vi "Read.Lookup.vi"(8 "error in (no error)":errorcluster, 10 "Name":string, 11 "Data Access API in":refnum<class "Data Access Engine.lvclass">) -> (0 "error out":errorcluster, 1 "Found?":bool, 2 "Ref":refnum<data-value>, 3 "Data Access API out":refnum<class "Data Access Engine.lvclass">)   [LabVIEW 2015, in "Data Access Engine.lvlib" / "Data Access Engine.lvclass"]
uses:
  Data Access Engine.lvclass
  Data/Read/Read.lvclass
  Data Access Engine.lvclass/Data Access Engine.ctl
  Types/VS Channel Group Type.ctl
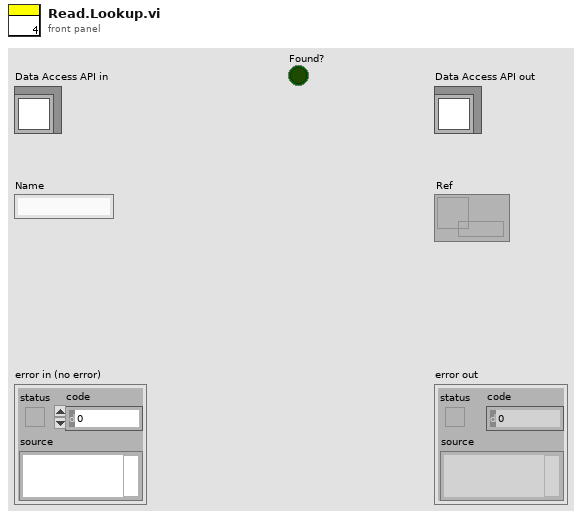
[diagram p1: front panel]
types:
  T1 = typedef "Data Access Engine.lvlib/Data Access Engine.lvclass/VS Channel Group Type.ctl" = enum16{"Output/Write", "Input/Read", "Input/ReadWrite"}
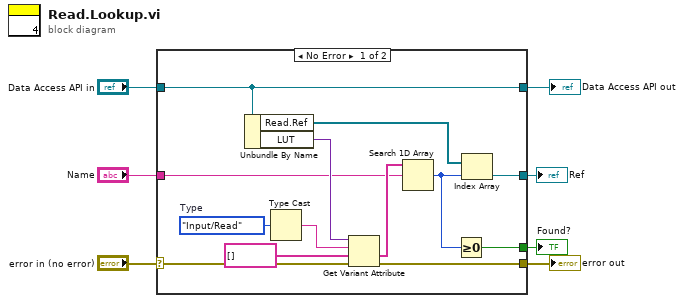
[diagram p0: block diagram]
diagram:
  n1 = case shown="No Error" "error in (no error)" {
    selector: "error in (no error)" -> [w16 w22]
    tunnel: [w15 w22] -> w6
    tunnel: [w20 w21] -> w4
    tunnel: "Data Access API in" -> [w20 w21]
    tunnel: "Name" -> [w13 _]
    tunnel: [w11 _] -> w2
    tunnel: [w9 _] -> w1
    frame No Error {
      w8 = VS_Channel_Group_Type."Input/Read"  # Type
      n2 = Unbundle By Name(w20) -> ("Read.Ref"=w12:refnum<data-value>[], "LUT"=w19:variant)
      n3 = Type Cast(x=w8) -> (*(type *) &x=w18:string)  [unwired: 1 in]
      n4 = Get Variant Attribute(Variant=w19, name=w18, default value (empty Variant)=string[] [], error in=w16) -> (value=w14:string[], error out=w15:errorcluster)  [unwired: 2 out]
      n5 = Search 1D Array(1D array=w14, element=w13) -> (index of element=w10:i32)  [unwired: 1 in]
      n6 = Greater Or Equal To 0?(x=w10) -> (x >= 0?=w9:bool)
      n7 = Index Array(array=w12, index=w10) -> (element=w11:refnum<data-value>)
    }
    frame Error {
    }
  }
  "error out" <- w6
  "Data Access API out" <- w4
  "Ref" <- w2
  "Found?" <- w1
